vi "ShowMSG.vi"(8 "error in (no error)":errorcluster, 10 "String":string, 11 "First Actor in":refnum<class "First Actor.lvclass">) -> (0 "error out":errorcluster, 3 "First Actor out":refnum<class "First Actor.lvclass">)   [LabVIEW 2020, in "First Actor.lvlib" / "First Actor.lvclass"]
uses:
  First Actor.lvclass
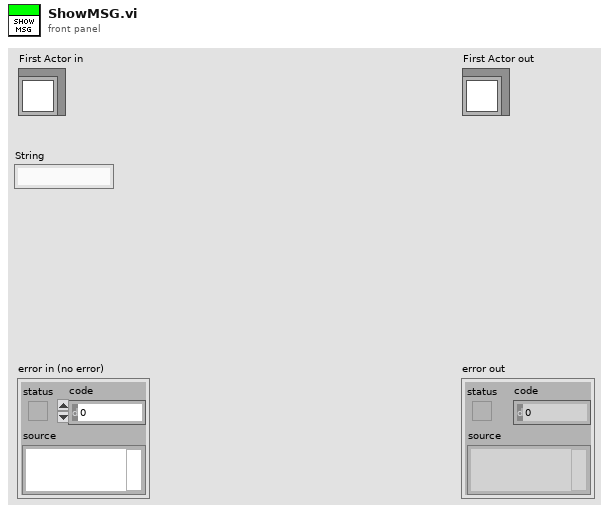
[diagram p1: front panel]
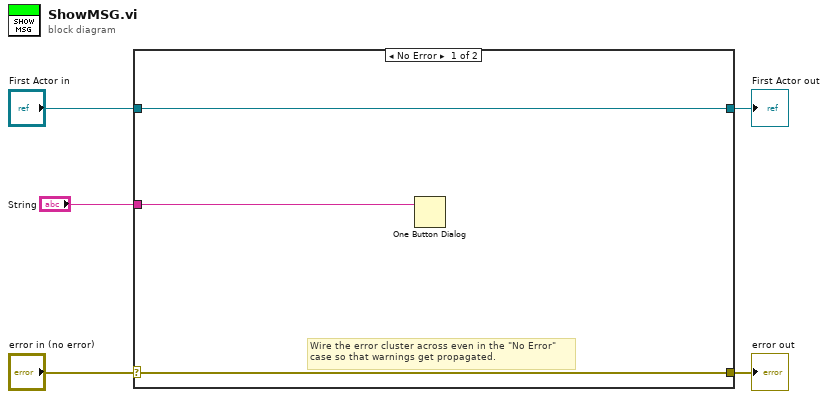
[diagram p0: block diagram]
diagram:
  n1 = case shown="No Error" "error in (no error)" {
    selector: "error in (no error)" -> [w7 w10]
    tunnel: [w7 w10] -> w4
    tunnel: [w8 w9] -> w2
    tunnel: "First Actor in" -> [w8 w9]
    tunnel: "String" -> [w6 _]
    frame No Error {
      # "Wire the error cluster across even in the \"No Error\"\ncase so that warnings get propagated."
      n2 = One Button Dialog(message=w6) -> ()  [unwired: 1 in, 1 out]
    }
    frame Error {
    }
  }
  "error out" <- w4
  "First Actor out" <- w2
